vi "DVL_2_QUAD (SubVI).vi"(11 "dvl_m":dbl[](array[numeric])) -> (0 "DVL OK":bool[](array[boolean]), 2 "dvl_sig":i32[](array[numeric]), 3 "DVL":dbl[](array[numeric]))   [LabVIEW 2014]
uses:
  <vilib>/imath/engines/lvmath2/RunTimeEngine/RangeToken/NIMS_Range_R2 - Integer.vi
  <instcachedir>/0/NIMS_Range_R2 - Integer_2D1304BAF97744E0A293025746CBADFC.lvgen/NIMS_Range_R2 - Integer_2D1304BAF97744E0A293025746CBADFC_000.vi
  <vilib>/imath/engines/lvmath2/RunTimeEngine/CommandStatement/MC_CommandStatement_break.vi
  <vilib>/imath/engines/lvmath2/RunTimeEngine/IndexRead/NIMS V(S).vi
  <instcachedir>/0/NIMS V(S)_0488751826AF41519A22953C041130DC.lvgen/NIMS V(S)_0488751826AF41519A22953C041130DC_000.vi
  <vilib>/imathl/engines/lvmath/Functions/Error Handling/Create Error.vi
  <vilib>/imath/engines/lvmath2/RunTimeEngine/IndexReplace/NIMS V(S)=S.vi
  <instcachedir>/0/NIMS V(S)=S_2D52C4EC15D8415E870AEE69FB516CCA.lvgen/NIMS V(S)=S_2D52C4EC15D8415E870AEE69FB516CCA_004.vi
  <vilib>/imath/engines/lvmath2/RunTimeEngine/NodeEndStatement/NIMS_NodeEndStatement_Output.vi
  <instcachedir>/0/NIMS_NodeEndStatement_Output_53EC0D466D134D7ABD903AC30B43404B.lvgen/NIMS_NodeEndStatement_Output_53EC0D466D134D7ABD903AC30B43404B_004.vi
  <vilib>/imath/engines/lvmath2/RunTimeEngine/ErrorHandling/NIMS_Finalize Error.vi
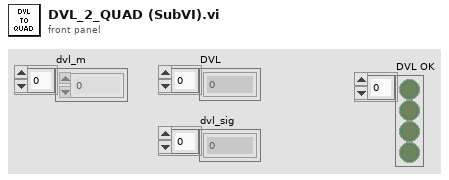
[diagram p1: front panel]
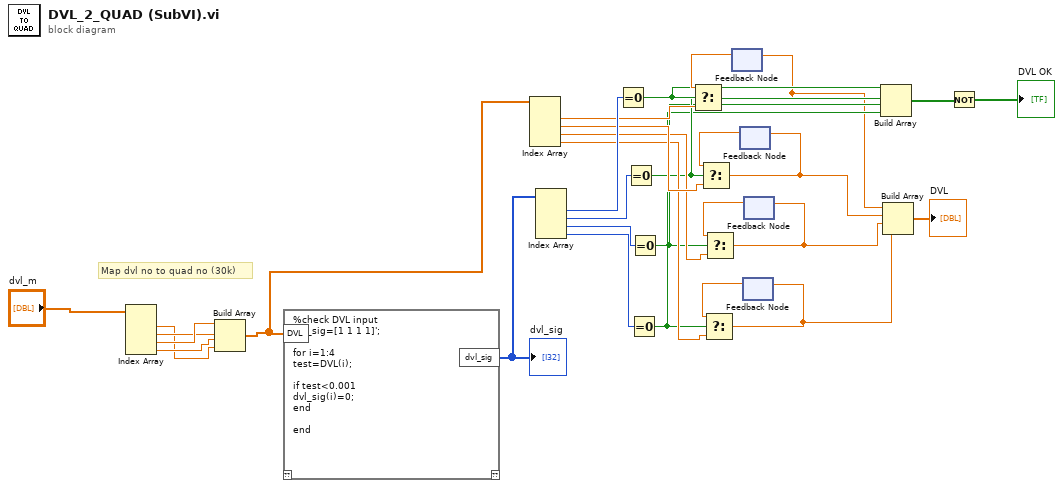
[diagram p0: block diagram]
diagram:
  # "Map dvl no to quad no (30k)"
  n1 = Index Array(array="dvl_m") -> (element #1=w1:dbl, element #2=w3:dbl, element #3=w4:dbl, element #4=w2:dbl)  [unwired: 4 in]
  n2 = Build Array(w4, w3, w2, w1) -> (w8:dbl[])
  n3 = mathscript code="%check DVL input\ndvl_sig=[1 1 1 1]';\n\nfor i=1:4\ntest=DVL(i);\n\nif test<0.001\ndvl_sig(i)=0;\nend\n\nend"("DVL"=w8) -> ("dvl_sig"=w28:i32[])  [unwired: 1 in, 1 out]
  "dvl_sig" <- w28
  n4 = Index Array(array=w8) -> (element #1=w26:dbl, element #2=w19:dbl, element #3=w18:dbl, element #4=w17:dbl)  [unwired: 4 in]
  n5 = Index Array(array=w28) -> (element #1=w27:i32, element #2=w22:i32, element #3=w21:i32, element #4=w20:i32)  [unwired: 4 in]
  n6 = Equal To 0?(x=w27) -> (x = 0?=w16:bool)
  n7 = Equal To 0?(x=w22) -> (x = 0?=w15:bool)
  n8 = Equal To 0?(x=w20) -> (x = 0?=w13:bool)
  n9 = Equal To 0?(x=w21) -> (x = 0?=w14:bool)
  n10 = feedback #1() -> (w29:dbl)  [unwired: 1 in]
  n11 = Select(t=w29, s=w16, f=w26) -> (s? t:f=w12:dbl)
  n12 = feedback-in #1(w12) -> ()
  n13 = feedback #2() -> (w25:dbl)  [unwired: 1 in]
  n14 = Select(t=w25, s=w15, f=w19) -> (s? t:f=w11:dbl)
  n15 = feedback-in #2(w11) -> ()
  n16 = feedback #3() -> (w23:dbl)  [unwired: 1 in]
  n17 = Select(t=w23, s=w13, f=w17) -> (s? t:f=w9:dbl)
  n18 = feedback-in #3(w9) -> ()
  n19 = feedback #4() -> (w24:dbl)  [unwired: 1 in]
  n20 = Select(t=w24, s=w14, f=w18) -> (s? t:f=w10:dbl)
  n21 = feedback-in #4(w10) -> ()
  n22 = Build Array(w16, w15, w14, w13) -> (w6:bool[])
  n23 = Build Array(w12, w11, w10, w9) -> (→"DVL":dbl[])
  n24 = Not(x=w6) -> (.not. x?=→"DVL OK":bool[])
